vi "When Test Case Has Parent - Adds Entire Hierarchy.vi"() -> ()   [LabVIEW 2017, in "ResultTree.Tests.lvlib" / "Add Tests.lvlib"]
uses:
  Add Tests.lvlib
  ef84827f-beff-4aab-89a2-e12a28173cfa.vi
  Constraint/IsEqual/Create.vi
  Constraint/IsEqual/IsEqual.lvclass
  ResultTree/ResultTree.lvclass
  Test Case/Test Case.lvclass
panel:
  out "error out":errorcluster
  in  "Tree":string(tree)
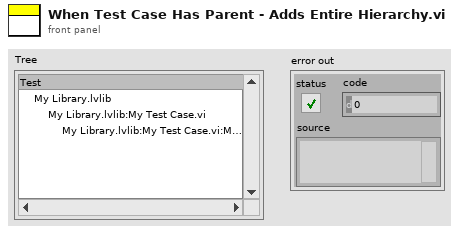
[diagram p1: front panel]
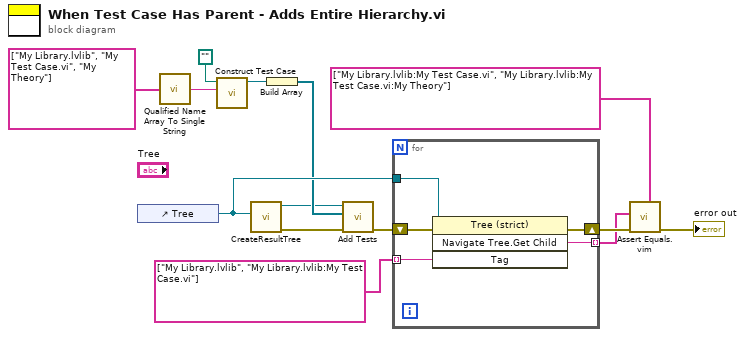
[diagram p0: block diagram]
diagram:
  n1 = control-ref of="Tree"() -> (w13:refnum<vi>)
  n2 = call <vilib>:"Qualified Name Array To Single String.vi"("Fully Qualified Array"=string[] ["My Library.lvlib", "My Test Case.vi", "My Theory"]) -> ("Fully Qualified String"=w7:string)
  n3 = call "Construct Test Case.vi"("Qualified Name"=w7, "Path"=path "") -> ("Test Case"=w3:refnum<class "Test Case.lvclass">)  [unwired: 8 in, 1 out]
  n4 = call "CreateResultTree.vi"("Tree Refnum"=w13) -> ("error out"=w6:errorcluster, "ResultTree out"=w1:refnum<class "ResultTree.lvclass">)  [unwired: 9 in]
  n5 = Build Array(w3) -> (w2:refnum<class "Test Case.lvclass">[])
  n6 = call "Add Tests.vi"("error in (no error)"=w6, "Test Cases"=w2, "ResultTree in"=w1) -> ("error out"=w10:errorcluster)  [unwired: 7 in, 1 out]
  n7 = for {
    tunnel: w13 -> [w19]
    tunnel: string[] ["My Library.lvlib", "My Library.lvlib:My Test Case.vi"] ("Name") -> [w17] mode=indexing
    shift-right: [w18] -> w12
    shift-left: w10 -> [w16]
    tunnel: [w15] -> w5 mode=indexing
    n8 = invoke class="Tree (strict)" method="Navigate Tree.Get Child"(reference=w19, error in=w16, "Tag"=w17) -> (error out=w18:errorcluster, "Navigate Tree:Get Child"=w15:string)  [unwired: 1 in, 2 out]
  }
  n9 = call "Assert Equals.vim"("Expected"=string[] ["My Library.lvlib:My Test Case.vi", "My Library.lvlib:My Test Case.vi:My Theory"] ("Name"), "error in (no error)"=w12, "Actual"=w5) -> ("error out"=→"error out":errorcluster)  [unwired: 8 in]
